vi "配置通信参数.vi"(8 "error in (no error)":errorcluster, 10 "通信设置输入":cluster{"本地端口":u16, "最大字节数/读取":i32}, 11 "串口通信类 in":refnum<class "串口通信类.lvclass">) -> (0 "error out":errorcluster, 3 "串口通信类 out":refnum<class "串口通信类.lvclass">)   [LabVIEW 2015, in "串口通信类.lvclass"]
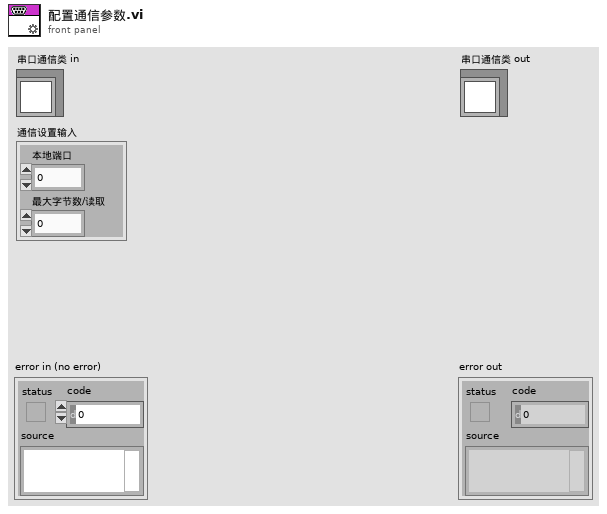
[diagram p1: front panel]
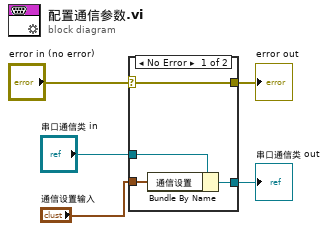
[diagram p0: block diagram]
diagram:
  n1 = case shown="No Error" "error in (no error)" {
    selector: "error in (no error)" -> [w6 w11]
    tunnel: "串口通信类 in" -> [w9 w10]
    tunnel: "通信设置输入" -> [w8 _]
    tunnel: [w7 w10] -> w3
    tunnel: [w6 w11] -> w1
    frame No Error {
      n2 = Bundle By Name(cluster=w9, "通信设置"=w8) -> (w7:refnum<class "串口通信类.lvclass">)
    }
    frame Error {
    }
  }
  "error out" <- w1
  "串口通信类 out" <- w3
